vi "Dave.vi"() -> ()   [LabVIEW 2013]
panel:
  out "String":string
  out "Dave":u16(ring)
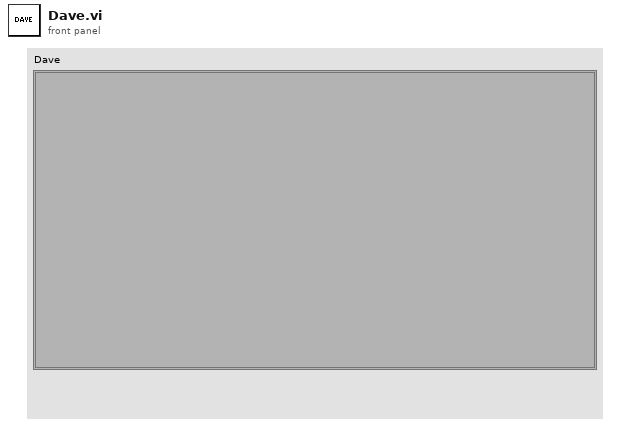
[diagram p1: front panel]
types:
  T1 = enum32{"Invalid", "Standard", "Closed", "Hidden", "Minimized", "Maximized"}
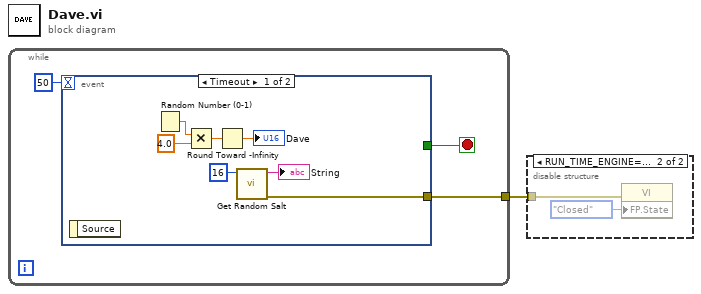
[diagram p0: block diagram]
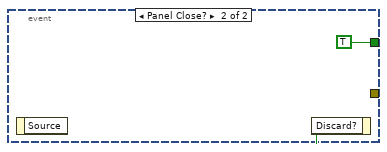
[diagram p3: hidden frame]
diagram:
  n1 = while {
    tunnel: [w2] -> w1
    stop <- w4 stop-if-true
    n2 = event shown="[0] Timeout" {
      selector: _ -> [_ _]
      dyn-events: _ -> [_ _]
      timeout: 50 -> [_ _]
      tunnel: [_ TRUE] -> w4
      tunnel: [w5 _] -> w2
      event Timeout {
        n3 = event-data() -> ()  [unwired: 1 in, 1 out]
        n4 = Random Number (0-1)() -> (number: 0 to 1=w10:dbl)
        n5 = Multiply(x=w10, y=4.0) -> (x*y=w8:dbl)
        n6 = Round Toward -Infinity(1:w8) -> (0:→"Dave":dbl)
        n7 = call "Get Random Salt.vi"("# of bytes (32)"=16) -> ("error out"=w5:errorcluster, "hex salt"=→"String":string)  [unwired: 8 in, 1 out]
      }
      event Panel Close? {
        n8 = event-data() -> ()  [unwired: 1 in, 1 out]
        n9 = event-data("Discard?"=TRUE) -> ()  [unwired: 1 in, 1 out]
      }
    }
  }
  n10 = disable-structure shown="RUN_TIME_ENGINE==True" {
    disable-tunnel: w1 -> [_ w15]
    frame condition #0 (active) {
    }
    frame condition #1 {
      n11 = property class="VI"(error in=w15, "FP.State"=T1."Closed" ("Front Panel Window:State")) -> ()  [unwired: 1 in, 2 out]
    }
  }
